vi "select_sample_port.vi"(1 "counter-clockwise?":bool, 2 "wait for ready to return?":bool=TRUE, 3 "Sample Port":u16(ring) items=["A"=1, "B"=2, "C"=3, "D"=4, "E"=5, "F"=6, "G"=7, "H"=8], 4 "kloehn session in":T1={"VISA resource out"="COM12", "error out"={"status"=FALSE, "code"=0, "source"=""}}) -> (0 "kloehn session out":T1={"VISA resource out"="COM12", "error out"={"status"=FALSE, "code"=0, "source"=""}})   [LabVIEW 2010]
panel:
  # "Later, this VI should be rewritten in order to make selection of a new port quicker (by knowing whether clockwise or counter clockwise is going to be fastest)."
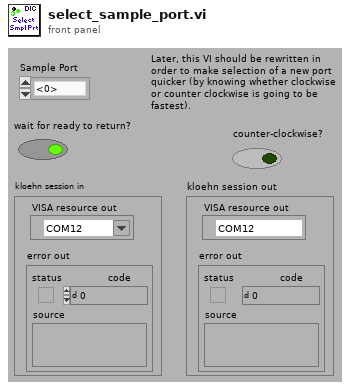
[diagram p1: front panel]
types:
  T1 = cluster{"VISA resource out":refnum<visa-resource-name>, "error out":errorcluster}
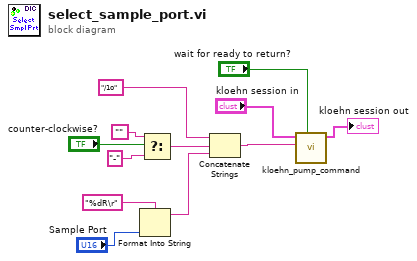
[diagram p0: block diagram]
diagram:
  n1 = Format Into String(format string="%dR\r", "Sample Port") -> (resulting string=w3:string)  [unwired: 2 in, 1 out]
  n2 = Select(t="", s="counter-clockwise?", f="-") -> (s? t:f=w2:string)
  n3 = Concatenate Strings("/1o", w2, w3) -> (w9:string)
  n4 = call "kloehn_pump_command.vi"("wait for ready to return?"="wait for ready to return?", "Send String"=w9, "kloehn session in"="kloehn session in") -> ("kloehn session out"=→"kloehn session out":T1)  [unwired: 5 in, 3 out]
